vi "SetDriveCurrent.vi"(2 "Current":sgl, 3 "Device":u8=1, 4 "Serial port":refnum<visa-resource-name>) -> (0 "Device out":u8=1, 1 "Serial port out":refnum<visa-resource-name>)   [LabVIEW 2021]
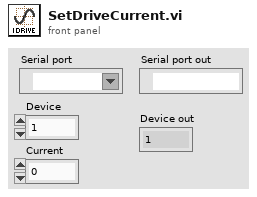
[diagram p1: front panel]
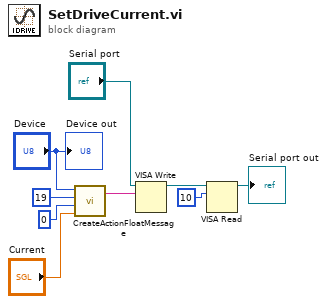
[diagram p0: block diagram]
diagram:
  n1 = call "CreateActionFloatMessage.vi"("Value"="Current", "Key"=u32 0, "Action"=u8 19, "Device"="Device") -> ("Message"=w2:string)  [unwired: 1 in]
  n2 = VISA Write(VISA resource name="Serial port", write buffer=w2) -> (VISA resource name out=w9:refnum<visa-resource-name>)  [unwired: 1 in, 2 out]
  n3 = VISA Read(VISA resource name=w9, byte count=u32 10) -> (VISA resource name out=→"Serial port out":refnum<visa-resource-name>)  [unwired: 1 in, 3 out]
  "Device out" <- "Device"
